vi "Write Full Computation.vi"(8 "error in (no error)":errorcluster, 10 "Full Computation?":bool, 11 "Video Processor in":refnum<class "Video Processor.lvclass">) -> (0 "error out":errorcluster, 3 "Video Processor out":refnum<class "Video Processor.lvclass">)   [LabVIEW 2018, in "Video Processor.lvclass"]
uses:
  Video Processor.lvclass
  Video Processor.lvclass/Video Processor.ctl
  Roughness Averager/Roughness Averager.lvclass
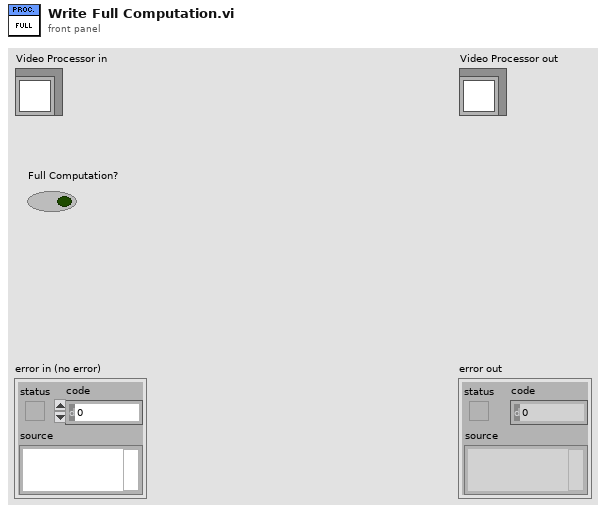
[diagram p1: front panel]
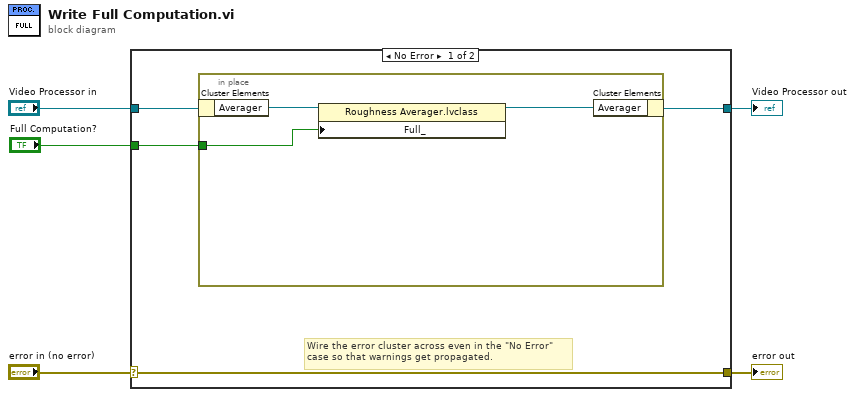
[diagram p0: block diagram]
diagram:
  n1 = case shown="No Error" "error in (no error)" {
    selector: "error in (no error)" -> [w9 w14]
    tunnel: [w9 w14] -> w4
    tunnel: [w6 w13] -> w2
    tunnel: "Video Processor in" -> [w8 w13]
    tunnel: "Full Computation?" -> [w7 _]
    frame No Error {
      # "Wire the error cluster across even in the \"No Error\"\ncase so that warnings get propagated."
      n2 = in-place {
        in-place-border: w7 -> [w11]
        n3 = in-place-cluster #1(w8) -> ("Averager"=w12:refnum<class "Roughness Averager.lvclass">)
        n4 = property class="Roughness Averager.lvclass"(reference=w12, "Full_"=w11) -> (reference out=w10:refnum<class "Roughness Averager.lvclass">)  [unwired: 1 in, 1 out]
        n5 = in-place-cluster #1("Averager"=w10) -> (w6:refnum<class "Video Processor.lvclass">)
      }
    }
    frame Error {
    }
  }
  "error out" <- w4
  "Video Processor out" <- w2
